vi "诊断标定3 - 副本.vi"(8 "CAN端口":u16(ring), 9 "设备索引号":u16(ring), 10 "CAN卡类型":u32(ring)=21) -> ()   [LabVIEW 2013] (continued)
                n1427 = Index Array(array=w1884) -> (element #3=w1874:bool, element #4=w1873:bool, element #5=w1872:bool, element #6=w1871:bool, element #7=w1870:bool, element #8=w1869:bool)  [unwired: 8 in, 2 out]
                n1428 = Index Array(array=w1885) -> (element #3=w1883:bool, element #4=w1882:bool, element #5=w1881:bool, element #6=w1880:bool, element #7=w1879:bool, element #8=w1878:bool)  [unwired: 8 in, 2 out]
                n1429 = Build Array(w1874, w1873, w1872, w1871, w1870, w1869) -> (w1875:bool[])
                n1430 = Build Array(w1883, w1882, w1881, w1880, w1879, w1878) -> (w1877:bool[])
                n1431 = And Array Elements(Boolean array=w1875) -> (logical AND=w1868:bool)
                n1432 = And Array Elements(Boolean array=w1877) -> (logical AND=w1876:bool)
                n1433 = Not(x=w1867) -> (.not. x?=w1891:bool)
              }
              frame "电池包信息1" {
                w1896 = 2
                w1904 = 2
                w1895 = 2
                w1893 = FALSE ("1 6")
                n1434 = Select(t=0, s=w1901, f=1) -> (s? t:f=w1894:i32)
                n1435 = property on="串联数" class="DigNum (严格)"("Disabled"=w1894) -> ()  [unwired: 2 in, 2 out]
                n1436 = property on="并联数" class="DigNum (严格)"("Disabled"=w1894) -> ()  [unwired: 2 in, 2 out]
                n1437 = property on="电池厂家" class="DigNum (严格)"("Disabled"=w1894) -> ()  [unwired: 2 in, 2 out]
                n1438 = property on="电池类型" class="DigNum (严格)"("Disabled"=w1894) -> ()  [unwired: 2 in, 2 out]
                n1439 = property on="额定能量" class="DigNum (严格)"("Disabled"=w1894) -> ()  [unwired: 2 in, 2 out]
                n1440 = property on="额定容量" class="DigNum (严格)"("Disabled"=w1894) -> ()  [unwired: 2 in, 2 out]
                n1441 = property on="实际容量" class="DigNum (严格)"("Disabled"=w1894) -> ()  [unwired: 2 in, 2 out]
                n1442 = property on="电池组信息" class="Clust (严格)"("Disabled"=w1894) -> ()  [unwired: 2 in, 2 out]
                n1443 = property on="生产日期" class="Str"("DisabledEnum"=w1894) -> ()  [unwired: 2 in, 2 out]
                n1444 = property on="车牌号" class="Str"("DisabledEnum"=w1895) -> ()  [unwired: 2 in, 2 out]
                n1445 = property on="产权标识" class="DigNum (严格)"("Disabled"=w1894) -> ()  [unwired: 2 in, 2 out]
                n1446 = property on="应用车型" class="DigNum (严格)"("Disabled"=w1894) -> ()  [unwired: 2 in, 2 out]
                n1447 = property on="额定总压" class="DigNum (严格)"("Disabled"=w1894) -> ()  [unwired: 2 in, 2 out]
                n1448 = property on="电池包序号" class="DigNum (严格)"("DisabledEnum"=w1894) -> ()  [unwired: 2 in, 2 out]
                n1449 = property on="电池包组号" class="DigNum (严格)"("DisabledEnum"=w1895) -> ()  [unwired: 2 in, 2 out]
                n1450 = property on="最大允许单体电压" class="DigNum (严格)"("Disabled"=w1904) -> ()  [unwired: 2 in, 2 out]
                n1451 = property on="最大允许总电压" class="DigNum (严格)"("Disabled"=w1904) -> ()  [unwired: 2 in, 2 out]
                n1452 = property on="最大允许温度" class="DigNum (严格)"("Disabled"=w1904) -> ()  [unwired: 2 in, 2 out]
                n1453 = property on="最小允许温度" class="DigNum (严格)"("Disabled"=w1904) -> ()  [unwired: 2 in, 2 out]
                n1454 = property on="最大允许充电电流" class="DigNum (严格)"("Disabled"=w1904) -> ()  [unwired: 2 in, 2 out]
                n1455 = property on="最小允许充电电流" class="DigNum (严格)"("Disabled"=w1904) -> ()  [unwired: 2 in, 2 out]
                n1456 = property on="最小允许单体电压" class="DigNum (严格)"("Disabled"=w1904) -> ()  [unwired: 2 in, 2 out]
                n1457 = property on="电流步长" class="DigNum (严格)"("Disabled"=w1904) -> ()  [unwired: 2 in, 2 out]
                n1458 = property on="SOC" class="DigNum (严格)"("Disabled"=w1904) -> ()  [unwired: 2 in, 2 out]
                n1459 = property on="充电总安时" class="DigNum (严格)"("Disabled"=w1904) -> ()  [unwired: 2 in, 2 out]
                n1460 = property on="放电总安时" class="DigNum (严格)"("Disabled"=w1904) -> ()  [unwired: 2 in, 2 out]
                n1461 = property on="放空次数" class="DigNum (严格)"("DisabledEnum"=w1896) -> ()  [unwired: 2 in, 2 out]
                n1462 = property on="充满次数" class="DigNum (严格)"("DisabledEnum"=w1896) -> ()  [unwired: 2 in, 2 out]
                n1463 = property on="充电次数" class="DigNum (严格)"("DisabledEnum"=w1896) -> ()  [unwired: 2 in, 2 out]
                n1464 = global read "功能码全局.vi" "24"() -> (w1899:bool[])
                n1465 = global read "功能码全局.vi" "23"() -> (w1900:bool[])
                n1466 = Index Array(array=w1899) -> (element #3=w1897:bool)  [unwired: 8 in, 7 out]
                n1467 = Index Array(array=w1900) -> (element #3=w1898:bool)  [unwired: 8 in, 7 out]
                n1468 = Not(x=w1893) -> (.not. x?=w1905:bool)
              }
              frame "电池包组号" {
                w1910 = 2
                w1909 = 2
                w1919 = 2
                w1911 = 2
                w1920 = 2
                w1907 = FALSE ("1 6")
                n1469 = property on="串联数" class="DigNum (严格)"("Disabled"=w1920) -> ()  [unwired: 2 in, 2 out]
                n1470 = property on="并联数" class="DigNum (严格)"("Disabled"=w1920) -> ()  [unwired: 2 in, 2 out]
                n1471 = property on="电池厂家" class="DigNum (严格)"("Disabled"=w1920) -> ()  [unwired: 2 in, 2 out]
                n1472 = property on="电池类型" class="DigNum (严格)"("Disabled"=w1920) -> ()  [unwired: 2 in, 2 out]
                n1473 = property on="额定能量" class="DigNum (严格)"("Disabled"=w1920) -> ()  [unwired: 2 in, 2 out]
                n1474 = property on="额定容量" class="DigNum (严格)"("Disabled"=w1920) -> ()  [unwired: 2 in, 2 out]
                n1475 = property on="实际容量" class="DigNum (严格)"("Disabled"=w1920) -> ()  [unwired: 2 in, 2 out]
                n1476 = Select(t=0, s=w1916, f=1) -> (s? t:f=w1908:i32)
                n1477 = property on="生产日期" class="Str"("DisabledEnum"=w1910) -> ()  [unwired: 2 in, 2 out]
                n1478 = property on="电池包序号" class="DigNum (严格)"("DisabledEnum"=w1910) -> ()  [unwired: 2 in, 2 out]
                n1479 = property on="车牌号" class="Str"("DisabledEnum"=w1910) -> ()  [unwired: 2 in, 2 out]
                n1480 = property on="电池包组号" class="DigNum (严格)"("DisabledEnum"=w1908) -> ()  [unwired: 2 in, 2 out]
                n1481 = property on="电池组信息" class="Clust (严格)"("Disabled"=w1908) -> ()  [unwired: 2 in, 2 out]
                n1482 = property on="产权标识" class="DigNum (严格)"("Disabled"=w1911) -> ()  [unwired: 2 in, 2 out]
                n1483 = property on="应用车型" class="DigNum (严格)"("Disabled"=w1911) -> ()  [unwired: 2 in, 2 out]
                n1484 = property on="额定总压" class="DigNum (严格)"("Disabled"=w1911) -> ()  [unwired: 2 in, 2 out]
                n1485 = property on="放空次数" class="DigNum (严格)"("DisabledEnum"=w1909) -> ()  [unwired: 2 in, 2 out]
                n1486 = property on="充满次数" class="DigNum (严格)"("DisabledEnum"=w1909) -> ()  [unwired: 2 in, 2 out]
                n1487 = property on="充电次数" class="DigNum (严格)"("DisabledEnum"=w1909) -> ()  [unwired: 2 in, 2 out]
                n1488 = property on="最大允许单体电压" class="DigNum (严格)"("Disabled"=w1919) -> ()  [unwired: 2 in, 2 out]
                n1489 = property on="最大允许总电压" class="DigNum (严格)"("Disabled"=w1919) -> ()  [unwired: 2 in, 2 out]
                n1490 = property on="最大允许温度" class="DigNum (严格)"("Disabled"=w1919) -> ()  [unwired: 2 in, 2 out]
                n1491 = property on="最小允许温度" class="DigNum (严格)"("Disabled"=w1919) -> ()  [unwired: 2 in, 2 out]
                n1492 = property on="最大允许充电电流" class="DigNum (严格)"("Disabled"=w1919) -> ()  [unwired: 2 in, 2 out]
                n1493 = property on="最小允许充电电流" class="DigNum (严格)"("Disabled"=w1919) -> ()  [unwired: 2 in, 2 out]
                n1494 = property on="最小允许单体电压" class="DigNum (严格)"("Disabled"=w1919) -> ()  [unwired: 2 in, 2 out]
                n1495 = property on="电流步长" class="DigNum (严格)"("Disabled"=w1919) -> ()  [unwired: 2 in, 2 out]
                n1496 = property on="SOC" class="DigNum (严格)"("Disabled"=w1919) -> ()  [unwired: 2 in, 2 out]
                n1497 = property on="充电总安时" class="DigNum (严格)"("Disabled"=w1919) -> ()  [unwired: 2 in, 2 out]
                n1498 = property on="放电总安时" class="DigNum (严格)"("Disabled"=w1919) -> ()  [unwired: 2 in, 2 out]
                n1499 = global read "功能码全局.vi" "24"() -> (w1914:bool[])
                n1500 = global read "功能码全局.vi" "23"() -> (w1915:bool[])
                n1501 = Index Array(array=w1914) -> (element #3=w1912:bool)  [unwired: 8 in, 7 out]
                n1502 = Index Array(array=w1915) -> (element #3=w1913:bool)  [unwired: 8 in, 7 out]
                n1503 = Not(x=w1907) -> (.not. x?=w1921:bool)
              }
              frame "充放电安时" {
                w1925 = 2
                w1924 = 2
                w1934 = 2
                w1935 = 2
                w1937 = 2
                w1923 = FALSE ("1 6")
                n1504 = property on="串联数" class="DigNum (严格)"("Disabled"=w1937) -> ()  [unwired: 2 in, 2 out]
                n1505 = property on="并联数" class="DigNum (严格)"("Disabled"=w1937) -> ()  [unwired: 2 in, 2 out]
                n1506 = property on="电池厂家" class="DigNum (严格)"("Disabled"=w1937) -> ()  [unwired: 2 in, 2 out]
                n1507 = property on="电池类型" class="DigNum (严格)"("Disabled"=w1937) -> ()  [unwired: 2 in, 2 out]
                n1508 = property on="额定能量" class="DigNum (严格)"("Disabled"=w1937) -> ()  [unwired: 2 in, 2 out]
                n1509 = property on="额定容量" class="DigNum (严格)"("Disabled"=w1937) -> ()  [unwired: 2 in, 2 out]
                n1510 = property on="实际容量" class="DigNum (严格)"("Disabled"=w1937) -> ()  [unwired: 2 in, 2 out]
                n1511 = Select(t=0, s=w1931, f=1) -> (s? t:f=w1930:i32)
                n1512 = property on="生产日期" class="Str"("DisabledEnum"=w1925) -> ()  [unwired: 2 in, 2 out]
                n1513 = property on="电池包序号" class="DigNum (严格)"("DisabledEnum"=w1925) -> ()  [unwired: 2 in, 2 out]
                n1514 = property on="车牌号" class="Str"("DisabledEnum"=w1925) -> ()  [unwired: 2 in, 2 out]
                n1515 = property on="电池包组号" class="DigNum (严格)"("DisabledEnum"=w1925) -> ()  [unwired: 2 in, 2 out]
                n1516 = property on="电池组信息" class="Clust (严格)"("Disabled"=w1930) -> ()  [unwired: 2 in, 2 out]
                n1517 = property on="额定总压" class="DigNum (严格)"("Disabled"=2) -> ()  [unwired: 2 in, 2 out]
                n1518 = property on="产权标识" class="DigNum (严格)"("Disabled"=w1935) -> ()  [unwired: 2 in, 2 out]
                n1519 = property on="应用车型" class="DigNum (严格)"("Disabled"=w1935) -> ()  [unwired: 2 in, 2 out]
                n1520 = property on="放空次数" class="DigNum (严格)"("DisabledEnum"=w1924) -> ()  [unwired: 2 in, 2 out]
                n1521 = property on="充满次数" class="DigNum (严格)"("DisabledEnum"=w1924) -> ()  [unwired: 2 in, 2 out]
                n1522 = property on="充电次数" class="DigNum (严格)"("DisabledEnum"=w1924) -> ()  [unwired: 2 in, 2 out]
                n1523 = property on="最大允许单体电压" class="DigNum (严格)"("Disabled"=w1934) -> ()  [unwired: 2 in, 2 out]
                n1524 = property on="最大允许总电压" class="DigNum (严格)"("Disabled"=w1934) -> ()  [unwired: 2 in, 2 out]
                n1525 = property on="最大允许温度" class="DigNum (严格)"("Disabled"=w1934) -> ()  [unwired: 2 in, 2 out]
                n1526 = property on="最小允许温度" class="DigNum (严格)"("Disabled"=w1934) -> ()  [unwired: 2 in, 2 out]
                n1527 = property on="最大允许充电电流" class="DigNum (严格)"("Disabled"=w1934) -> ()  [unwired: 2 in, 2 out]
                n1528 = property on="最小允许充电电流" class="DigNum (严格)"("Disabled"=w1934) -> ()  [unwired: 2 in, 2 out]
                n1529 = property on="最小允许单体电压" class="DigNum (严格)"("Disabled"=w1934) -> ()  [unwired: 2 in, 2 out]
                n1530 = property on="电流步长" class="DigNum (严格)"("Disabled"=w1934) -> ()  [unwired: 2 in, 2 out]
                n1531 = property on="SOC" class="DigNum (严格)"("Disabled"=w1934) -> ()  [unwired: 2 in, 2 out]
                n1532 = property on="充电总安时" class="DigNum (严格)"("Disabled"=w1930) -> ()  [unwired: 2 in, 2 out]
                n1533 = property on="放电总安时" class="DigNum (严格)"("Disabled"=w1930) -> ()  [unwired: 2 in, 2 out]
                n1534 = Not(x=w1923) -> (.not. x?=w1938:bool)
                n1535 = global read "功能码全局.vi" "24"() -> (w1928:bool[])
                n1536 = global read "功能码全局.vi" "23"() -> (w1929:bool[])
                n1537 = Index Array(array=w1928) -> (element #7=w1926:bool)  [unwired: 8 in, 7 out]
                n1538 = Index Array(array=w1929) -> (element #7=w1927:bool)  [unwired: 8 in, 7 out]
              }
              frame "充电次数" {
                w1943 = 2
                w1952 = 2
                w1953 = 2
                w1944 = 2
                w1954 = 2
                w1940 = FALSE ("1 6")
                n1539 = property on="串联数" class="DigNum (严格)"("Disabled"=w1954) -> ()  [unwired: 2 in, 2 out]
                n1540 = property on="并联数" class="DigNum (严格)"("Disabled"=w1954) -> ()  [unwired: 2 in, 2 out]
                n1541 = property on="电池厂家" class="DigNum (严格)"("Disabled"=w1954) -> ()  [unwired: 2 in, 2 out]
                n1542 = property on="电池类型" class="DigNum (严格)"("Disabled"=w1954) -> ()  [unwired: 2 in, 2 out]
                n1543 = property on="额定能量" class="DigNum (严格)"("Disabled"=w1954) -> ()  [unwired: 2 in, 2 out]
                n1544 = property on="额定容量" class="DigNum (严格)"("Disabled"=w1954) -> ()  [unwired: 2 in, 2 out]
                n1545 = property on="实际容量" class="DigNum (严格)"("Disabled"=w1954) -> ()  [unwired: 2 in, 2 out]
                n1546 = Select(t=0, s=w1949, f=1) -> (s? t:f=w1941:i32)
                n1547 = property on="生产日期" class="Str"("DisabledEnum"=w1943) -> ()  [unwired: 2 in, 2 out]
                n1548 = property on="电池包序号" class="DigNum (严格)"("DisabledEnum"=w1943) -> ()  [unwired: 2 in, 2 out]
                n1549 = property on="车牌号" class="Str"("DisabledEnum"=w1943) -> ()  [unwired: 2 in, 2 out]
                n1550 = property on="电池组信息" class="Clust (严格)"("Disabled"=w1941) -> ()  [unwired: 2 in, 2 out]
                n1551 = property on="电池包组号" class="DigNum (严格)"("DisabledEnum"=w1943) -> ()  [unwired: 2 in, 2 out]
                n1552 = property on="额定总压" class="DigNum (严格)"("Disabled"=w1944) -> ()  [unwired: 2 in, 2 out]
                n1553 = property on="产权标识" class="DigNum (严格)"("Disabled"=w1944) -> ()  [unwired: 2 in, 2 out]
                n1554 = property on="应用车型" class="DigNum (严格)"("Disabled"=w1944) -> ()  [unwired: 2 in, 2 out]
                n1555 = property on="放空次数" class="DigNum (严格)"("DisabledEnum"=w1941) -> (error out=w1942:errorcluster)  [unwired: 2 in, 1 out]
                n1556 = property on="充满次数" class="DigNum (严格)"("DisabledEnum"=w1941) -> ()  [unwired: 2 in, 2 out]
                n1557 = property on="充电次数" class="DigNum (严格)"("DisabledEnum"=w1941) -> ()  [unwired: 2 in, 2 out]
                n1558 = property on="最大允许单体电压" class="DigNum (严格)"("Disabled"=w1953) -> ()  [unwired: 2 in, 2 out]
                n1559 = property on="最大允许总电压" class="DigNum (严格)"("Disabled"=w1953) -> ()  [unwired: 2 in, 2 out]
                n1560 = property on="最大允许温度" class="DigNum (严格)"("Disabled"=w1953) -> ()  [unwired: 2 in, 2 out]
                n1561 = property on="最小允许温度" class="DigNum (严格)"("Disabled"=w1953) -> ()  [unwired: 2 in, 2 out]
                n1562 = property on="最大允许充电电流" class="DigNum (严格)"("Disabled"=w1953) -> ()  [unwired: 2 in, 2 out]
                n1563 = property on="最小允许充电电流" class="DigNum (严格)"(error in=w1942, "Disabled"=w1953) -> ()  [unwired: 1 in, 2 out]
                n1564 = property on="最小允许单体电压" class="DigNum (严格)"("Disabled"=w1953) -> ()  [unwired: 2 in, 2 out]
                n1565 = property on="电流步长" class="DigNum (严格)"("Disabled"=w1953) -> ()  [unwired: 2 in, 2 out]
                n1566 = property on="SOC" class="DigNum (严格)"("Disabled"=w1953) -> ()  [unwired: 2 in, 2 out]
                n1567 = property on="充电总安时" class="DigNum (严格)"("Disabled"=w1952) -> ()  [unwired: 2 in, 2 out]
                n1568 = property on="放电总安时" class="DigNum (严格)"("Disabled"=w1952) -> ()  [unwired: 2 in, 2 out]
                n1569 = Not(x=w1940) -> (.not. x?=w1955:bool)
                n1570 = global read "功能码全局.vi" "24"() -> (w1947:bool[])
                n1571 = global read "功能码全局.vi" "23"() -> (w1948:bool[])
                n1572 = Index Array(array=w1947) -> (element #8=w1946:bool)  [unwired: 8 in, 7 out]
                n1573 = Index Array(array=w1948) -> (element #8=w1945:bool)  [unwired: 8 in, 7 out]
              }
              frame "SOC" {
                w1959 = 2
                w1958 = 2
                w1968 = 2
                w1969 = 2
                w1970 = 2
                w1972 = 2
                w1957 = FALSE ("1 6")
                n1574 = property on="串联数" class="DigNum (严格)"("Disabled"=w1972) -> ()  [unwired: 2 in, 2 out]
                n1575 = property on="并联数" class="DigNum (严格)"("Disabled"=w1972) -> ()  [unwired: 2 in, 2 out]
                n1576 = property on="电池厂家" class="DigNum (严格)"("Disabled"=w1972) -> ()  [unwired: 2 in, 2 out]
                n1577 = property on="电池类型" class="DigNum (严格)"("Disabled"=w1972) -> ()  [unwired: 2 in, 2 out]
                n1578 = property on="额定能量" class="DigNum (严格)"("Disabled"=w1972) -> ()  [unwired: 2 in, 2 out]
                n1579 = property on="额定容量" class="DigNum (严格)"("Disabled"=w1972) -> ()  [unwired: 2 in, 2 out]
                n1580 = property on="实际容量" class="DigNum (严格)"("Disabled"=w1972) -> ()  [unwired: 2 in, 2 out]
                n1581 = Select(t=0, s=w1965, f=1) -> (s? t:f=w1964:i32)
                n1582 = property on="生产日期" class="Str"("DisabledEnum"=w1959) -> ()  [unwired: 2 in, 2 out]
                n1583 = property on="电池包序号" class="DigNum (严格)"("DisabledEnum"=w1959) -> ()  [unwired: 2 in, 2 out]
                n1584 = property on="车牌号" class="Str"("DisabledEnum"=w1959) -> ()  [unwired: 2 in, 2 out]
                n1585 = property on="电池包组号" class="DigNum (严格)"("DisabledEnum"=w1959) -> ()  [unwired: 2 in, 2 out]
                n1586 = property on="电池组信息" class="Clust (严格)"("Disabled"=w1964) -> ()  [unwired: 2 in, 2 out]
                n1587 = property on="SOC" class="DigNum (严格)"("Disabled"=w1964) -> ()  [unwired: 2 in, 2 out]
                n1588 = property on="额定总压" class="DigNum (严格)"("Disabled"=2) -> ()  [unwired: 2 in, 2 out]
                n1589 = property on="产权标识" class="DigNum (严格)"("Disabled"=w1970) -> ()  [unwired: 2 in, 2 out]
                n1590 = property on="应用车型" class="DigNum (严格)"("Disabled"=w1970) -> ()  [unwired: 2 in, 2 out]
                n1591 = property on="放空次数" class="DigNum (严格)"("DisabledEnum"=w1958) -> ()  [unwired: 2 in, 2 out]
                n1592 = property on="充满次数" class="DigNum (严格)"("DisabledEnum"=w1958) -> ()  [unwired: 2 in, 2 out]
                n1593 = property on="充电次数" class="DigNum (严格)"("DisabledEnum"=w1958) -> ()  [unwired: 2 in, 2 out]
                n1594 = property on="最大允许单体电压" class="DigNum (严格)"("Disabled"=w1969) -> ()  [unwired: 2 in, 2 out]
                n1595 = property on="最大允许总电压" class="DigNum (严格)"("Disabled"=w1969) -> ()  [unwired: 2 in, 2 out]
                n1596 = property on="最大允许温度" class="DigNum (严格)"("Disabled"=w1969) -> ()  [unwired: 2 in, 2 out]
                n1597 = property on="最小允许温度" class="DigNum (严格)"("Disabled"=w1969) -> ()  [unwired: 2 in, 2 out]
                n1598 = property on="最大允许充电电流" class="DigNum (严格)"("Disabled"=w1969) -> ()  [unwired: 2 in, 2 out]
                n1599 = property on="最小允许充电电流" class="DigNum (严格)"("Disabled"=w1969) -> ()  [unwired: 2 in, 2 out]
                n1600 = property on="最小允许单体电压" class="DigNum (严格)"("Disabled"=w1969) -> ()  [unwired: 2 in, 2 out]
                n1601 = property on="电流步长" class="DigNum (严格)"("Disabled"=w1969) -> ()  [unwired: 2 in, 2 out]
                n1602 = property on="充电总安时" class="DigNum (严格)"("Disabled"=w1968) -> ()  [unwired: 2 in, 2 out]
                n1603 = property on="放电总安时" class="DigNum (严格)"("Disabled"=w1968) -> ()  [unwired: 2 in, 2 out]
                n1604 = Not(x=w1957) -> (.not. x?=w1973:bool)
                n1605 = global read "功能码全局.vi" "24"() -> (w1962:bool[])
                n1606 = global read "功能码全局.vi" "23"() -> (w1963:bool[])
                n1607 = Index Array(array=w1962) -> (element #6=w1961:bool)  [unwired: 8 in, 7 out]
                n1608 = Index Array(array=w1963) -> (element #6=w1960:bool)  [unwired: 8 in, 7 out]
              }
              frame "车牌号" {
                w1978 = 2
                w1977 = 2
                w1987 = 2
                w1988 = 2
                w1989 = 2
                w1991 = 2
                w1975 = FALSE ("1 6")
                n1609 = property on="串联数" class="DigNum (严格)"("Disabled"=w1991) -> ()  [unwired: 2 in, 2 out]
                n1610 = property on="并联数" class="DigNum (严格)"("Disabled"=w1991) -> ()  [unwired: 2 in, 2 out]
                n1611 = property on="电池厂家" class="DigNum (严格)"("Disabled"=w1991) -> ()  [unwired: 2 in, 2 out]
                n1612 = property on="电池类型" class="DigNum (严格)"("Disabled"=w1991) -> ()  [unwired: 2 in, 2 out]
                n1613 = property on="额定能量" class="DigNum (严格)"("Disabled"=w1991) -> ()  [unwired: 2 in, 2 out]
                n1614 = property on="额定容量" class="DigNum (严格)"("Disabled"=w1991) -> ()  [unwired: 2 in, 2 out]
                n1615 = property on="实际容量" class="DigNum (严格)"("Disabled"=w1991) -> ()  [unwired: 2 in, 2 out]
                n1616 = Select(t=0, s=w1983, f=1) -> (s? t:f=w1976:i32)
                n1617 = property on="生产日期" class="Str"("DisabledEnum"=w1978) -> ()  [unwired: 2 in, 2 out]
                n1618 = property on="电池包序号" class="DigNum (严格)"("DisabledEnum"=w1978) -> ()  [unwired: 2 in, 2 out]
                n1619 = property on="电池包组号" class="DigNum (严格)"("DisabledEnum"=w1978) -> ()  [unwired: 2 in, 2 out]
                n1620 = property on="电池组信息" class="Clust (严格)"("Disabled"=w1976) -> ()  [unwired: 2 in, 2 out]
                n1621 = property on="车牌号" class="Str"("DisabledEnum"=w1976) -> ()  [unwired: 2 in, 2 out]
                n1622 = property on="额定总压" class="DigNum (严格)"("Disabled"=2) -> ()  [unwired: 2 in, 2 out]
                n1623 = property on="产权标识" class="DigNum (严格)"("Disabled"=w1989) -> ()  [unwired: 2 in, 2 out]
                n1624 = property on="应用车型" class="DigNum (严格)"("Disabled"=w1989) -> ()  [unwired: 2 in, 2 out]
                n1625 = property on="放空次数" class="DigNum (严格)"("DisabledEnum"=w1977) -> ()  [unwired: 2 in, 2 out]
                n1626 = property on="充满次数" class="DigNum (严格)"("DisabledEnum"=w1977) -> ()  [unwired: 2 in, 2 out]
                n1627 = property on="充电次数" class="DigNum (严格)"("DisabledEnum"=w1977) -> ()  [unwired: 2 in, 2 out]
                n1628 = property on="最大允许单体电压" class="DigNum (严格)"("Disabled"=w1988) -> ()  [unwired: 2 in, 2 out]
                n1629 = property on="最大允许总电压" class="DigNum (严格)"("Disabled"=w1988) -> ()  [unwired: 2 in, 2 out]
                n1630 = property on="最大允许温度" class="DigNum (严格)"("Disabled"=w1988) -> ()  [unwired: 2 in, 2 out]
                n1631 = property on="最小允许温度" class="DigNum (严格)"("Disabled"=w1988) -> ()  [unwired: 2 in, 2 out]
                n1632 = property on="最大允许充电电流" class="DigNum (严格)"("Disabled"=w1988) -> ()  [unwired: 2 in, 2 out]
                n1633 = property on="最小允许充电电流" class="DigNum (严格)"("Disabled"=w1988) -> ()  [unwired: 2 in, 2 out]
                n1634 = property on="最小允许单体电压" class="DigNum (严格)"("Disabled"=w1988) -> ()  [unwired: 2 in, 2 out]
                n1635 = property on="电流步长" class="DigNum (严格)"("Disabled"=w1988) -> ()  [unwired: 2 in, 2 out]
                n1636 = property on="SOC" class="DigNum (严格)"("Disabled"=2) -> ()  [unwired: 2 in, 2 out]
                n1637 = property on="充电总安时" class="DigNum (严格)"("Disabled"=w1987) -> ()  [unwired: 2 in, 2 out]
                n1638 = property on="放电总安时" class="DigNum (严格)"("Disabled"=w1987) -> ()  [unwired: 2 in, 2 out]
                n1639 = Not(x=w1975) -> (.not. x?=w1992:bool)
                n1640 = global read "功能码全局.vi" "24"() -> (w1981:bool[])
                n1641 = global read "功能码全局.vi" "23"() -> (w1982:bool[])
                n1642 = Index Array(array=w1981) -> (element #5=w1979:bool)  [unwired: 8 in, 7 out]
                n1643 = Index Array(array=w1982) -> (element #5=w1980:bool)  [unwired: 8 in, 7 out]
              }
              frame "充电参数" {
                w1996 = 2
                w1995 = 2
                w2005 = 2
                w2006 = 2
                w2008 = 2
                w1994 = FALSE ("1 6")
                n1644 = property on="串联数" class="DigNum (严格)"("Disabled"=w2008) -> ()  [unwired: 2 in, 2 out]
                n1645 = property on="并联数" class="DigNum (严格)"("Disabled"=w2008) -> ()  [unwired: 2 in, 2 out]
                n1646 = property on="电池厂家" class="DigNum (严格)"("Disabled"=w2008) -> ()  [unwired: 2 in, 2 out]
                n1647 = property on="电池类型" class="DigNum (严格)"("Disabled"=w2008) -> ()  [unwired: 2 in, 2 out]
                n1648 = property on="额定能量" class="DigNum (严格)"("Disabled"=w2008) -> ()  [unwired: 2 in, 2 out]
                n1649 = property on="额定容量" class="DigNum (严格)"("Disabled"=w2008) -> ()  [unwired: 2 in, 2 out]
                n1650 = property on="实际容量" class="DigNum (严格)"("Disabled"=w2008) -> ()  [unwired: 2 in, 2 out]
                n1651 = Select(t=0, s=w2002, f=1) -> (s? t:f=w2001:i32)
                n1652 = property on="生产日期" class="Str"("DisabledEnum"=w1996) -> ()  [unwired: 2 in, 2 out]
                n1653 = property on="电池包序号" class="DigNum (严格)"("DisabledEnum"=w1996) -> ()  [unwired: 2 in, 2 out]
                n1654 = property on="车牌号" class="Str"("DisabledEnum"=w1996) -> ()  [unwired: 2 in, 2 out]
                n1655 = property on="电池组信息" class="Clust (严格)"("Disabled"=w2001) -> ()  [unwired: 2 in, 2 out]
                n1656 = property on="电池包组号" class="DigNum (严格)"("DisabledEnum"=w1996) -> ()  [unwired: 2 in, 2 out]
                n1657 = property on="额定总压" class="DigNum (严格)"("Disabled"=2) -> ()  [unwired: 2 in, 2 out]
                n1658 = property on="产权标识" class="DigNum (严格)"("Disabled"=w2006) -> ()  [unwired: 2 in, 2 out]
                n1659 = property on="应用车型" class="DigNum (严格)"("Disabled"=w2006) -> ()  [unwired: 2 in, 2 out]
                n1660 = property on="放空次数" class="DigNum (严格)"("DisabledEnum"=w1995) -> ()  [unwired: 2 in, 2 out]
                n1661 = property on="充满次数" class="DigNum (严格)"("DisabledEnum"=w1995) -> ()  [unwired: 2 in, 2 out]
                n1662 = property on="充电次数" class="DigNum (严格)"("DisabledEnum"=w1995) -> ()  [unwired: 2 in, 2 out]
                n1663 = property on="最大允许单体电压" class="DigNum (严格)"("Disabled"=w2001) -> ()  [unwired: 2 in, 2 out]
                n1664 = property on="最大允许总电压" class="DigNum (严格)"("Disabled"=w2001) -> ()  [unwired: 2 in, 2 out]
                n1665 = property on="最大允许温度" class="DigNum (严格)"("Disabled"=w2001) -> ()  [unwired: 2 in, 2 out]
                n1666 = property on="最小允许温度" class="DigNum (严格)"("Disabled"=w2001) -> ()  [unwired: 2 in, 2 out]
                n1667 = property on="最大允许充电电流" class="DigNum (严格)"("Disabled"=w2001) -> ()  [unwired: 2 in, 2 out]
                n1668 = property on="最小允许充电电流" class="DigNum (严格)"("Disabled"=w2001) -> ()  [unwired: 2 in, 2 out]
                n1669 = property on="最小允许单体电压" class="DigNum (严格)"("Disabled"=w2001) -> ()  [unwired: 2 in, 2 out]
                n1670 = property on="电流步长" class="DigNum (严格)"("Disabled"=w2001) -> ()  [unwired: 2 in, 2 out]
                n1671 = property on="SOC" class="DigNum (严格)"("Disabled"=w2005) -> ()  [unwired: 2 in, 2 out]
                n1672 = property on="充电总安时" class="DigNum (严格)"("Disabled"=w2005) -> ()  [unwired: 2 in, 2 out]
                n1673 = property on="放电总安时" class="DigNum (严格)"("Disabled"=w2005) -> ()  [unwired: 2 in, 2 out]
                n1674 = Not(x=w1994) -> (.not. x?=w2009:bool)
                n1675 = global read "功能码全局.vi" "24"() -> (w1999:bool[])
                n1676 = global read "功能码全局.vi" "23"() -> (w2000:bool[])
                n1677 = Index Array(array=w1999) -> (element #4=w1997:bool)  [unwired: 8 in, 7 out]
                n1678 = Index Array(array=w2000) -> (element #4=w1998:bool)  [unwired: 8 in, 7 out]
              }
              frame "均衡参数" {
                w2011 = FALSE ("1 6")
                n1679 = Select(t=0, s=w2017, f=1) -> (s? t:f=w2015:i32)
                n1680 = property on="均衡计算-电压高阀值1级" class="DigNum (严格)"("DisabledEnum"=w2015) -> ()  [unwired: 2 in, 2 out]
                n1681 = property on="均衡计算-电压高阀值2级" class="DigNum (严格)"("DisabledEnum"=w2015) -> ()  [unwired: 2 in, 2 out]
                n1682 = property on="均衡计算-电压低阀值1级" class="DigNum (严格)"("DisabledEnum"=w2015) -> ()  [unwired: 2 in, 2 out]
                n1683 = property on="均衡计算-电压低阀值2级" class="DigNum (严格)"("DisabledEnum"=w2015) -> ()  [unwired: 2 in, 2 out]
                n1684 = property on="均衡计算-最低电压阀值" class="DigNum (严格)"("DisabledEnum"=w2015) -> ()  [unwired: 2 in, 2 out]
                n1685 = property on="均衡停止-最低电压阀值" class="DigNum (严格)"("DisabledEnum"=w2015) -> ()  [unwired: 2 in, 2 out]
                n1686 = property on="均衡计算-电压极差阀值" class="DigNum (严格)"("DisabledEnum"=w2015) -> ()  [unwired: 2 in, 2 out]
                n1687 = property on="均衡参数" class="Clust (严格)"("DisabledEnum"=w2015) -> ()  [unwired: 2 in, 2 out]
                n1688 = property on="充电结束电压(90%)" class="DigNum (严格)"("DisabledEnum"=w2015) -> ()  [unwired: 2 in, 2 out]
                n1689 = property on="充电结束电压(91%)" class="DigNum (严格)"("DisabledEnum"=w2015) -> ()  [unwired: 2 in, 2 out]
                n1690 = property on="充电结束电压(92%)" class="DigNum (严格)"("DisabledEnum"=w2015) -> ()  [unwired: 2 in, 2 out]
                n1691 = property on="充电结束电压(93%)" class="DigNum (严格)"("DisabledEnum"=w2015) -> ()  [unwired: 2 in, 2 out]
                n1692 = property on="充电结束电压(94%)" class="DigNum (严格)"("DisabledEnum"=w2015) -> ()  [unwired: 2 in, 2 out]
                n1693 = property on="充电结束电压(95%)" class="DigNum (严格)"("DisabledEnum"=w2015) -> ()  [unwired: 2 in, 2 out]
                n1694 = property on="充电结束电压(96%)" class="DigNum (严格)"("DisabledEnum"=w2015) -> ()  [unwired: 2 in, 2 out]
                n1695 = property on="充电结束电压(97%)" class="DigNum (严格)"("DisabledEnum"=w2015) -> ()  [unwired: 2 in, 2 out]
                n1696 = property on="充电结束电压(98%)" class="DigNum (严格)"("DisabledEnum"=w2015) -> ()  [unwired: 2 in, 2 out]
                n1697 = property on="充电结束电压(99%)" class="DigNum (严格)"("DisabledEnum"=w2015) -> ()  [unwired: 2 in, 2 out]
                n1698 = property on="充电结束电压(100%)" class="DigNum (严格)"("DisabledEnum"=w2015) -> ()  [unwired: 2 in, 2 out]
                n1699 = disable-structure shown="启用" {
                  disable-tunnel: [w2021 w2023] -> w2014
                  disable-tunnel: [w2020 w2023] -> w2013
                  frame Enabled {
                    n1700 = global read "功能码全局.vi" "18"() -> (w2022:bool[])
                    n1701 = Index Array(array=w2022) -> (element #1=w2021:bool, element #2=w2020:bool)  [unwired: 8 in, 6 out]
                  }
                  frame Disabled {
                    w2023 = TRUE
                  }
                }
                n1702 = Not(x=w2011) -> (.not. x?=w2012:bool)
              }
              frame "均衡阀值" {
                w2026 = 2
                w2024 = FALSE ("1 6")
                n1703 = Select(t=0, s=w2031, f=1) -> (s? t:f=w2029:i32)
                n1704 = property on="均衡计算-电压高阀值1级" class="DigNum (严格)"("DisabledEnum"=w2029) -> ()  [unwired: 2 in, 2 out]
                n1705 = property on="均衡计算-电压高阀值2级" class="DigNum (严格)"("DisabledEnum"=w2029) -> ()  [unwired: 2 in, 2 out]
                n1706 = property on="均衡计算-电压低阀值1级" class="DigNum (严格)"("DisabledEnum"=w2029) -> ()  [unwired: 2 in, 2 out]
                n1707 = property on="均衡计算-电压低阀值2级" class="DigNum (严格)"("DisabledEnum"=w2029) -> ()  [unwired: 2 in, 2 out]
                n1708 = property on="均衡计算-最低电压阀值" class="DigNum (严格)"("DisabledEnum"=w2029) -> ()  [unwired: 2 in, 2 out]
                n1709 = property on="均衡停止-最低电压阀值" class="DigNum (严格)"("DisabledEnum"=w2029) -> ()  [unwired: 2 in, 2 out]
                n1710 = property on="均衡计算-电压极差阀值" class="DigNum (严格)"("DisabledEnum"=w2029) -> ()  [unwired: 2 in, 2 out]
                n1711 = property on="均衡参数" class="Clust (严格)"("DisabledEnum"=w2029) -> ()  [unwired: 2 in, 2 out]
                n1712 = property on="充电结束电压(90%)" class="DigNum (严格)"("DisabledEnum"=w2026) -> ()  [unwired: 2 in, 2 out]
                n1713 = property on="充电结束电压(91%)" class="DigNum (严格)"("DisabledEnum"=w2026) -> ()  [unwired: 2 in, 2 out]
                n1714 = property on="充电结束电压(92%)" class="DigNum (严格)"("DisabledEnum"=w2026) -> ()  [unwired: 2 in, 2 out]
                n1715 = property on="充电结束电压(93%)" class="DigNum (严格)"("DisabledEnum"=w2026) -> ()  [unwired: 2 in, 2 out]
                n1716 = property on="充电结束电压(94%)" class="DigNum (严格)"("DisabledEnum"=w2026) -> ()  [unwired: 2 in, 2 out]
                n1717 = property on="充电结束电压(95%)" class="DigNum (严格)"("DisabledEnum"=w2026) -> ()  [unwired: 2 in, 2 out]
                n1718 = property on="充电结束电压(96%)" class="DigNum (严格)"("DisabledEnum"=w2026) -> ()  [unwired: 2 in, 2 out]
                n1719 = property on="充电结束电压(97%)" class="DigNum (严格)"("DisabledEnum"=w2026) -> ()  [unwired: 2 in, 2 out]
                n1720 = property on="充电结束电压(98%)" class="DigNum (严格)"("DisabledEnum"=w2026) -> ()  [unwired: 2 in, 2 out]
                n1721 = property on="充电结束电压(99%)" class="DigNum (严格)"("DisabledEnum"=w2026) -> ()  [unwired: 2 in, 2 out]
                n1722 = property on="充电结束电压(100%)" class="DigNum (严格)"("DisabledEnum"=w2026) -> ()  [unwired: 2 in, 2 out]
                n1723 = disable-structure shown="启用" {
                  disable-tunnel: [w2035 w2037] -> w2028
                  disable-tunnel: [w2034 w2037] -> w2027
                  frame Enabled {
                    n1724 = global read "功能码全局.vi" "18"() -> (w2036:bool[])
                    n1725 = Index Array(array=w2036) -> (element #1=w2035:bool, element #2=w2034:bool)  [unwired: 8 in, 6 out]
                  }
                  frame Disabled {
                    w2037 = TRUE
                  }
                }
                n1726 = Not(x=w2024) -> (.not. x?=w2025:bool)
              }
              frame "充电结束电压" {
                w2041 = 2
                w2038 = FALSE ("1 6")
                n1727 = Select(t=0, s=w2045, f=1) -> (s? t:f=w2040:i32)
                n1728 = property on="均衡计算-电压高阀值1级" class="DigNum (严格)"("DisabledEnum"=w2041) -> ()  [unwired: 2 in, 2 out]
                n1729 = property on="均衡计算-电压高阀值2级" class="DigNum (严格)"("DisabledEnum"=w2041) -> ()  [unwired: 2 in, 2 out]
                n1730 = property on="均衡计算-电压低阀值1级" class="DigNum (严格)"("DisabledEnum"=w2041) -> ()  [unwired: 2 in, 2 out]
                n1731 = property on="均衡计算-电压低阀值2级" class="DigNum (严格)"("DisabledEnum"=w2041) -> ()  [unwired: 2 in, 2 out]
                n1732 = property on="均衡计算-最低电压阀值" class="DigNum (严格)"("DisabledEnum"=w2041) -> ()  [unwired: 2 in, 2 out]
                n1733 = property on="均衡停止-最低电压阀值" class="DigNum (严格)"("DisabledEnum"=w2041) -> ()  [unwired: 2 in, 2 out]
                n1734 = property on="均衡计算-电压极差阀值" class="DigNum (严格)"("DisabledEnum"=w2041) -> ()  [unwired: 2 in, 2 out]
                n1735 = property on="均衡参数" class="Clust (严格)"("DisabledEnum"=w2040) -> ()  [unwired: 2 in, 2 out]
                n1736 = property on="充电结束电压(90%)" class="DigNum (严格)"("DisabledEnum"=w2040) -> ()  [unwired: 2 in, 2 out]
                n1737 = property on="充电结束电压(91%)" class="DigNum (严格)"("DisabledEnum"=w2040) -> ()  [unwired: 2 in, 2 out]
                n1738 = property on="充电结束电压(92%)" class="DigNum (严格)"("DisabledEnum"=w2040) -> ()  [unwired: 2 in, 2 out]
                n1739 = property on="充电结束电压(93%)" class="DigNum (严格)"("DisabledEnum"=w2040) -> ()  [unwired: 2 in, 2 out]
                n1740 = property on="充电结束电压(94%)" class="DigNum (严格)"("DisabledEnum"=w2040) -> ()  [unwired: 2 in, 2 out]
                n1741 = property on="充电结束电压(95%)" class="DigNum (严格)"("DisabledEnum"=w2040) -> ()  [unwired: 2 in, 2 out]
                n1742 = property on="充电结束电压(96%)" class="DigNum (严格)"("DisabledEnum"=w2040) -> ()  [unwired: 2 in, 2 out]
                n1743 = property on="充电结束电压(97%)" class="DigNum (严格)"("DisabledEnum"=w2040) -> ()  [unwired: 2 in, 2 out]
                n1744 = property on="充电结束电压(98%)" class="DigNum (严格)"("DisabledEnum"=w2040) -> ()  [unwired: 2 in, 2 out]
                n1745 = property on="充电结束电压(99%)" class="DigNum (严格)"("DisabledEnum"=w2040) -> ()  [unwired: 2 in, 2 out]
                n1746 = property on="充电结束电压(100%)" class="DigNum (严格)"("DisabledEnum"=w2040) -> ()  [unwired: 2 in, 2 out]
                n1747 = disable-structure shown="启用" {
                  disable-tunnel: [w2049 w2051] -> w2043
                  disable-tunnel: [w2048 w2051] -> w2042
                  frame Enabled {
                    n1748 = global read "功能码全局.vi" "18"() -> (w2050:bool[])
                    n1749 = Index Array(array=w2050) -> (element #1=w2049:bool, element #2=w2048:bool)  [unwired: 8 in, 6 out]
                  }
                  frame Disabled {
                    w2051 = TRUE
                  }
                }
                n1750 = Not(x=w2038) -> (.not. x?=w2039:bool)
              }
              frame "假", Default {
                w2052 = FALSE ("1 6")
                n1751 = Not(x=w2052) -> (.not. x?=w2053:bool)
              }
            }
            n1752 = local write "等级 2"(w1643) -> ()
            n1753 = local write "1 6"(w1642) -> ()
            n1754 = local write "1 7"(w1641) -> ()
            n1755 = local write "1 8"(w1640) -> ()
            n1756 = local write "1 9"(w1639) -> ()
            n1757 = local write "1 10"(w1638) -> ()
            n1758 = local write "1 12"(w1632) -> ()
            n1759 = property on="单个读取" class="Bool (严格)"("Visible"=w1637) -> ()  [unwired: 2 in, 2 out]
            n1760 = property on="单个写入" class="Bool (严格)"("Visible"=w1636) -> ()  [unwired: 2 in, 2 out]
          }
          event "从板个数": Value Change {
            n1761 = event-data() -> ()  [unwired: 7 out]
            n1762 = local read "从板个数"() -> (w2055:dbl)
            n1763 = call "多从板对应参数-new.vi"("从板个数"=w2055) -> ("输出数组"=w2056:string[])  [unwired: 1 in]
            n1764 = control-ref of="项目信息"() -> (w2057:refnum<vi>)
            n1765 = stacked-sequence {
              tunnel: w2057 -> [_ w2064 w2068]
              tunnel: w2056 -> [_ w2063 w2067]
              frame #0 {
                n1766 = local write "项目信息"(string[][] [] ("项目信息")) -> ()
              }
              frame #1 {
                n1767 = call "表格数据输入-8.6.vi"("行数"=u32 0, "列数"=u32 0, "字符串数组"=w2063, "表格引用"=w2064) -> ()  [unwired: 8 out]
              }
              frame #2 {
                n1768 = Array Size(array=w2067) -> (size(s)=w2066:i32)
                n1769 = for {
                  N: w2066 -> [_]
                  tunnel: [""] -> w2065 mode=indexing
                }
                n1770 = call "表格数据输入-8.6.vi"("行数"=u32 0, "列数"=u32 1, "字符串数组"=w2065, "表格引用"=w2068) -> ()  [unwired: 8 out]
              }
            }
          }
          event "主界面选项": Value Change {
            n1771 = event-data() -> ("NewVal"=w2072:enum32{"单选选项1", "单选选项2", "单选选项2 2", "单选选项2 3"})  [unwired: 6 out]
            n1772 = control-ref of="单选选项2 2"() -> (w2077:refnum<vi>)
            n1773 = control-ref of="单选选项2"() -> (w2079:refnum<vi>)
            n1774 = control-ref of="单选选项1"() -> (w2078:refnum<vi>)
            n1775 = control-ref of="单选选项2 3"() -> (w2073:refnum<vi>)
            n1776 = Build Array(w2078, w2079, w2077, w2073) -> (w2076:refnum<vi>[])
            n1777 = case shown="\"单选选项2 3\"" w2072 {
              selector: w2072 -> [w2090 w2095 w2100 w2105]
              tunnel: w2076 -> [w2091 w2096 w2101 w2106]
              tunnel: [w2089 w2094 w2099 w2104] -> w2082
              tunnel: [w2088 w2093 w2098 w2103] -> w2081
              tunnel: [enum32{"读写参数", "版本读取", "其它诊断"}."读写参数" ("选项卡控件 2") enum32{"读写参数", "版本读取", "其它诊断"}."版本读取" ("选项卡控件 2") enum32{"读写参数", "版本读取", "其它诊断"}."其它诊断" ("选项卡控件 2") enum32{"读写参数", "版本读取", "其它诊断", "高压板校正"}."高压板校正" ("选项卡控件 2")] -> w2080
              frame "单选选项1", Default {
                n1778 = Delete From Array(array=w2091, index=w2090) -> (deleted portion=w2088:refnum<vi>, array with subset deleted=w2089:refnum<vi>[])  [unwired: 1 in]
              }
              frame "单选选项2" {
                n1779 = Delete From Array(array=w2096, index=w2095) -> (deleted portion=w2093:refnum<vi>, array with subset deleted=w2094:refnum<vi>[])  [unwired: 1 in]
              }
              frame "单选选项2 2" {
                n1780 = Delete From Array(array=w2101, index=w2100) -> (deleted portion=w2098:refnum<vi>, array with subset deleted=w2099:refnum<vi>[])  [unwired: 1 in]
              }
              frame "单选选项2 3" {
                n1781 = Delete From Array(array=w2106, index=w2105) -> (deleted portion=w2103:refnum<vi>, array with subset deleted=w2104:refnum<vi>[])  [unwired: 1 in]
              }
            }
            n1782 = local write "面板选择"(w2080) -> ()
            n1783 = for {
              tunnel: u32 16777215 -> [w2086]
              tunnel: w2082 -> [w2085] mode=indexing
              n1784 = property class="Bool (严格)"(reference=w2085, "BoolText.TextColor"=w2086) -> ()  [unwired: 1 in, 2 out]
            }
            n1785 = property class="Bool (严格)"(reference=w2081, "BoolText.TextColor"=u32 65511) -> ()  [unwired: 1 in, 2 out]
          }
          event "主从板": Value Change {
            w2108 = FALSE ("可见")
            n1786 = event-data() -> ()  [unwired: 7 out]
            n1787 = control-ref of="单选选项2"() -> (w2116:refnum<vi>)
            n1788 = control-ref of="单选选项1"() -> (w2115:refnum<vi>)
            n1789 = local read "主从板"() -> (w2123:enum32{"单选选项2", "单选选项1"})
            n1790 = Build Array(w2116, w2115) -> (w2122:refnum<vi>[])
            n1791 = case shown="\"单选选项2\"" w2123 {
              selector: w2123 -> [w2168 w2211]
              tunnel: w2122 -> [w2169 w2210]
              tunnel: [enum32{"主板", "从板"}."主板" ("主从选择") enum32{"主板", "从板"}."从板" ("主从选择")] -> w2121
              tunnel: [w2167 w2209] -> w2118
              tunnel: [w2166 w2208] -> w2117
              tunnel: [TRUE FALSE] -> w2113
              tunnel: [w2127 w2188] -> w2110
              tunnel: [w2128 w2193] -> w2109
              tunnel: [FALSE ("可见") TRUE ("可见")] -> w2107
              frame "单选选项1", Default {
                n1792 = global read "功能码全局.vi" "主板项目信息7"() -> (w2139:bool[])
                n1793 = global read "功能码全局.vi" "主板项目信息4"() -> (w2162:bool[])
                n1794 = global read "功能码全局.vi" "主板控制类信息10"() -> (w2143:bool[])
                n1795 = global read "功能码全局.vi" "主板故障阀值9"() -> (w2140:bool[])
                n1796 = global read "功能码全局.vi" "主板项目信息5"() -> (w2153:bool[])
                n1797 = global read "功能码全局.vi" "主板项目信息6"() -> (w2163:bool[])
                n1798 = global read "功能码全局.vi" "主板版本号11"() -> (w2154:bool[])
                n1799 = Delete From Array(array=w2163, length=1 ("长度"), index=0 ("索引")) -> (deleted portion=w2152:bool[], array with subset deleted=w2135:bool[])
                n1800 = Index Array(array=w2162, index #1=5 ("索引"), index #2=6 ("索引")) -> (element #1=w2151:bool, element #2=w2134:bool)
                n1801 = Index Array(array=w2154) -> (element #1=w2147:bool, element #2=w2130:bool)  [unwired: 2 in]
                n1802 = Array Subset(array=w2140, index=2 ("索引"), length=3 ("长度")) -> (w2149:bool[])
                n1803 = Delete From Array(array=w2139, length=3 ("索引"), index=2 ("长度")) -> (deleted portion=w2150:bool[], array with subset deleted=w2133:bool[])
                n1804 = Array Subset(array=w2143, index=4 ("索引"), length=2 ("长度")) -> (w2148:bool[])
                n1805 = Delete From Array(array=w2169, index=w2168) -> (deleted portion=w2166:refnum<vi>, array with subset deleted=w2167:refnum<vi>[])  [unwired: 1 in]
                n1806 = Insert Into Array(array=w2153, new element #1=w2152, new element #2=w2151, new element #3=w2150, new element #4=w2149, new element #5=w2148, new element #6=w2147) -> (w2146:bool[])  [unwired: 1 in]
                n1807 = Array Subset(array=w2143, index=6 ("索引"), length=2 ("长度")) -> (w2131:bool[])
                n1808 = Array Subset(array=w2140, index=5 ("索引"), length=3 ("长度")) -> (w2132:bool[])
                n1809 = And Array Elements(Boolean array=w2146) -> (logical AND=w2128:bool)
                n1810 = Insert Into Array(array=w2135, new element #1=w2134, new element #2=w2133, new element #3=w2132, new element #4=w2131, new element #5=w2130) -> (w2129:bool[])  [unwired: 1 in]
                n1811 = And Array Elements(Boolean array=w2129) -> (logical AND=w2127:bool)
              }
              frame "单选选项2" {
                n1812 = global read "功能码全局.vi" "18"() -> (w2184:bool[])
                n1813 = global read "功能码全局.vi" "15"() -> (w2205:bool[])
                n1814 = global read "功能码全局.vi" "16"() -> (w2202:bool[])
                n1815 = Delete From Array(array=w2210, index=w2211) -> (deleted portion=w2208:refnum<vi>, array with subset deleted=w2209:refnum<vi>[])  [unwired: 1 in]
                n1816 = Index Array(array=w2202, index #1=4 ("索引"), index #2=5 ("索引"), index #3=6 ("索引"), index #4=7 ("索引")) -> (element #1=w2196:bool, element #2=w2195:bool, element #3=w2191:bool, element #4=w2190:bool)
                n1817 = Index Array(array=w2184, index #1=4 ("索引"), index #2=5 ("索引"), index #3=6 ("索引"), index #4=7 ("索引"), index #5=2 ("索引"), index #6=3 ("索引"), index #7=0 ("索引"), index #8=1 ("索引")) -> (element #1=w2177:bool, element #2=w2180:bool, element #3=w2179:bool, element #4=w2178:bool, element #5=w2176:bool, element #6=w2175:bool, element #7=w2170:bool, element #8=w2171:bool)
                n1818 = Delete From Array(array=w2205, length=4 ("长度"), index=0 ("索引")) -> (deleted portion=w2197:bool[], array with subset deleted=w2192:bool[])
                n1819 = Insert Into Array(array=w2192, new element #1=w2191, new element #2=w2190, new element #3=w2180, new element #4=w2179, new element #5=w2178, new element #6=w2171) -> (w2189:bool[])  [unwired: 1 in]
                n1820 = Insert Into Array(array=w2197, new element #1=w2196, new element #2=w2195, new element #3=w2177, new element #4=w2176, new element #5=w2175, new element #6=w2170) -> (w2194:bool[])  [unwired: 1 in]
                n1821 = And Array Elements(Boolean array=w2194) -> (logical AND=w2193:bool)
                n1822 = And Array Elements(Boolean array=w2189) -> (logical AND=w2188:bool)
              }
            }
            n1823 = property on="全部写入" class="Bool (严格)"("Visible"=w2110) -> ()  [unwired: 2 in, 2 out]
            n1824 = property on="全部读取" class="Bool (严格)"("Visible"=w2109) -> ()  [unwired: 2 in, 2 out]
            n1825 = property on="从板号" class="DigNum (严格)"("Visible"=w2107) -> ()  [unwired: 2 in, 2 out]
            n1826 = local write "主从选择"(w2121) -> ()
            n1827 = property on="从板个数" class="DigNum (严格)"("Visible"=w2113) -> ()  [unwired: 2 in, 2 out]
            n1828 = for {
              tunnel: u32 87470 -> [w2125]
              tunnel: w2118 -> [w2124] mode=indexing
              n1829 = property class="Bool (严格)"(reference=w2124, "BoolText.TextColor"=w2125) -> ()  [unwired: 1 in, 2 out]
            }
            n1830 = Not(x=w2113) -> (.not. x?=w2114:bool)
            n1831 = property class="Bool (严格)"(reference=w2117, "BoolText.TextColor"=u32 16777215) -> ()  [unwired: 1 in, 2 out]
            n1832 = property on="主板选项" class="Tree (严格)"("Visible"=w2113) -> ()  [unwired: 2 in, 2 out]
            n1833 = property on="从板选项" class="Tree (严格)"("Visible"=w2114) -> ()  [unwired: 2 in, 2 out]
            n1834 = property on="当前从板板号" class="DigNum (严格)"("Visible"=w2114) -> ()  [unwired: 2 in, 2 out]
            n1835 = property on="单个读取" class="Bool (严格)"("Visible"=w2108) -> ()  [unwired: 2 in, 2 out]
            n1836 = property on="单个写入" class="Bool (严格)"("Visible"=w2108) -> ()  [unwired: 2 in, 2 out]
          }
          event "从板号": Value Change {
            n1837 = event-data() -> ()  [unwired: 7 out]
            n1838 = local read "key names"() -> (w2213:string[])
            n1839 = Empty Array?(array=w2213) -> (empty?=w2212:bool)
            n1840 = case shown="假" w2212 {
              tunnel: w2213 -> [w2216 _]
              frame False {
                n1841 = stacked-sequence {
                  seq-local: [w2217 _] -> [_ w2280]
                  tunnel: w2216 -> [w2225 _]
                  frame #0 {
                    w2256 = 2 ("长度")
                    w2253 = 20 ("长度")
                    w2241 = 1 ("索引")
                    n1842 = local read "从板号"() -> (w2217:u8)
                    n1843 = local read "输出数组"() -> (w2226:string[][])
                    n1844 = Decrement(x=w2217) -> (x-1=w2223:u8)
                    n1845 = Index Array(array=w2226, index (col)=w2223) -> (element=w2254:string[])  [unwired: 1 in]
                    n1846 = global write "读配置文件全局2.vi" "从板板号"(w2217) -> ()
                    n1847 = Search 1D Array(1D array=w2225, element="风机开启温度" ("元素")) -> (index of element=w2238:i32)  [unwired: 1 in]
                    n1848 = Search 1D Array(1D array=w2225, element="电压过高一级" ("元素"), start index (0)=w2238) -> (index of element=w2236:i32)
                    n1849 = Decrement(x=w2238) -> (x-1=w2240:i32)
                    n1850 = Array Subset(array=w2254, index=w2241, length=w2240) -> (w2224:string[])
                    n1851 = Array Subset(array=w2254, index=w2236, length=21 ("长度")) -> (w2228:string[])
                    n1852 = Array Subset(array=w2225, index=w2241, length=w2240) -> (w2271:string[])
                    n1853 = Array Subset(array=w2254, index=w2238, length=7 ("长度")) -> (w2234:string[])
                    n1854 = for {
                      tunnel: w2228 -> [w2273] mode=indexing
                      tunnel: [w2272] -> w2227 mode=indexing
                      n1855 = Fract/Exp String To Number(string=w2273) -> (number=w2272:dbl)  [unwired: 3 in, 1 out]
                    }
                    n1856 = for {
                      tunnel: w2234 -> [w2275] mode=indexing
                      tunnel: [w2274] -> w2218 mode=indexing
                      n1857 = Fract/Exp String To Number(string=w2275) -> (number=w2274:dbl)  [unwired: 3 in, 1 out]
                    }
                    n1858 = Delete From Array(array=w2227, length=7 ("长度"), index=0 ("索引")) -> (deleted portion=w2221:dbl[], array with subset deleted=w2231:dbl[])
                    n1859 = Array To Cluster(array=w2218) -> (cluster=w2243:T20)
                    n1860 = global write "读配置文件全局2.vi" "加热控制参数"(w2218) -> ()
                    n1861 = Delete From Array(array=w2231, length=7 ("长度"), index=0 ("索引")) -> (deleted portion=w2220:dbl[], array with subset deleted=w2219:dbl[])
                    n1862 = local write "加热控制参数"(w2243) -> ()
                    n1863 = Array To Cluster(array=w2221) -> (cluster=w2268:T20)
                    n1864 = Array To Cluster(array=w2219) -> (cluster=w2270:T20)
                    n1865 = Array To Cluster(array=w2220) -> (cluster=w2269:T20)
                    n1866 = global write "读配置文件全局2.vi" "三级故障阀值"(w2219) -> ()
                    n1867 = global write "读配置文件全局2.vi" "一级故障阀值"(w2221) -> ()
                    n1868 = global write "读配置文件全局2.vi" "二级故障阀值"(w2220) -> ()
                    n1869 = local write "一级故障 6"(w2268) -> ()
                    n1870 = local write "一级故障 8"(w2270) -> ()
                    n1871 = local write "一级故障 7"(w2269) -> ()
                    n1872 = Search 1D Array(1D array=w2271, element="温度个数" ("元素")) -> (index of element=w2250:i32)  [unwired: 1 in]
                    n1873 = Search 1D Array(1D array=w2271, element="第一个保险通道" ("元素")) -> (index of element=w2251:i32)  [unwired: 1 in]
                    n1874 = Search 1D Array(1D array=w2271, element="电压个数" ("元素")) -> (index of element=w2249:i32)  [unwired: 1 in]
                    n1875 = Search 1D Array(1D array=w2271, element="第1通道电压个数" ("元素")) -> (index of element=w2252:i32)  [unwired: 1 in]
                    n1876 = Array Subset(array=w2224, index=w2249, length=2 ("长度")) -> (w2257:string[])
                    n1877 = Array Subset(array=w2224, index=w2250, length=w2256) -> (w2259:string[])
                    n1878 = Array Subset(array=w2224, index=w2251, length=20 ("长度")) -> (w2260:string[])
                    n1879 = Array Subset(array=w2224, index=w2252, length=w2253) -> (w2258:string[])
                    n1880 = Insert Into Array(array=w2257, new element #1=w2258, new element #2=w2259, new element #3=w2260) -> (w2222:string[])  [unwired: 1 in]
                    n1881 = Array Subset(array=w2271, index=w2249, length=w2256) -> (w2261:string[])
                    n1882 = Array Subset(array=w2271, index=w2250, length=w2256) -> (w2263:string[])
                    n1883 = Array Subset(array=w2271, index=w2251, length=w2253) -> (w2264:string[])
                    n1884 = Array Subset(array=w2271, index=w2252, length=w2253) -> (w2262:string[])
                    n1885 = global write "读配置文件全局2.vi" "表格"(w2222) -> ()
                    n1886 = Insert Into Array(array=w2261, new element #1=w2262, new element #2=w2263, new element #3=w2264) -> (w2266:string[])  [unwired: 1 in]
                    n1887 = Build Array(w2266, w2222) -> (w2265:string[][])
                    n1888 = Transpose 2D Array(2D array=w2265) -> (transposed array=w2267:string[][])
                    n1889 = local write "项目信息 2"(w2267) -> ()
                  }
                  frame #1 {
                    n1890 = Number To Decimal String(number=w2280) -> (decimal integer string=w2278:string)  [unwired: 1 in]
                    n1891 = control-ref of="结果"() -> (w2283:refnum<vi>)
                    n1892 = Concatenate Strings("从板", w2278, "导入完成") -> (w2276:string)
                    n1893 = Build Array(w2276) -> (w2281:string[])
                    n1894 = call "表格编辑.vi"("新元素/子数组"=w2281, "活动单元格:单元格背景色"=u32 6618880, "MCListbox引用句柄"=w2283) -> ()  [unwired: 9 out]
                  }
                }
              }
              frame True {
              }
            }
          }
          event "读配置文件": Value Change {
            n1895 = event-data() -> ("NewVal"=w2284:bool)  [unwired: 6 out]
            n1896 = case shown="真" w2284 {
              tunnel: w2288 -> [w2290 w2296]
              tunnel: [w2290 w2295] -> w2287
